vi "Anti-Tip.vi"() -> ()   [LabVIEW 2014]
uses:
  Begin/Global RefNums.vi
  Begin/Global Variables.vi
  _Dependencies/NavX/navX-MXP IMU.lvlib
panel:
  in  "Min Roll":dbl=-12.0
  in  "Min Pitch":dbl=-9.0
  in  "Max Roll":dbl=7.0
  in  "Max Pitch":dbl=6.0
  in  "Buffer":dbl=5.0
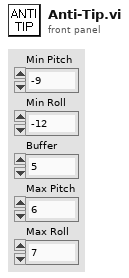
[diagram p1: front panel]
types:
  T1 = typedef "navX-MXP IMU.lvlib/navX Device TypeDef.ctl" = cluster{"navX Interface Protocol":T2, "navX Interface Protocol TypeDefs":cluster{"SPIDevRef":T3, "I2CDevRef":T6}, "navX System Information":cluster{"Board Information":T8, "Status":T9, "Offsets":T13}, "navX Common Information":cluster{"Update Rate (4Hz-60Hz)":T14, "refnum name":string, "error":errorcluster}}
  T2 = typedef "navX-MXP IMU.lvlib/navX Interface Protocol.ctl" = enum16{"SPI", "I2C"}
  T3 = typedef "WPI_SPIDevRef.ctl" = cluster{"DevStatus":errorcluster, "Handle":i32, "Controller":T4, "SPI Bus":T5}
  T4 = typedef "FPGA_TypedefDigitalModule.ctl" = enum16{"Controller 1"}
  T5 = typedef "spi_bus.ctl" = enum16{"SPI On-Board, CS0", "SPI On-Board, CS1", "SPI On-Board, CS2", "SPI On-Board, CS3", "SPI MXP", "Invalid"}
  T6 = typedef "WPI_I2CDevRef.ctl" = cluster{"DevStatus":errorcluster, "Controller":T4, "Device Address":u8, "Handle":i32, "I2C Bus":T7}
  T7 = typedef "i2c_bus.ctl" = enum16{"I2C On-Board", "I2C MXP", "Invalid"}
  T8 = typedef "navX-MXP IMU.lvlib/navX Board Information.ctl" = cluster{"WhoAmI (50 | 0x32)":u8, "Board Revision":u8, "Firmware Major Version":u8, "Firmware Minor Version":u8}
  T9 = typedef "navX-MXP IMU.lvlib/navX Status Data.ctl" = cluster{"Update Rate Hz":u8, "Accelerometer Full-Scale Range":u8, "Gyro Full-Scale Range":u16, "NAVX_OP_STATUS":T10, "NAVX_CAL_STATUS":T11, "NAVX_SELFTEST_STATUS":u8, "NAVX_SENSOR_STATUS":T12}
  T10 = typedef "navX-MXP IMU.lvlib/navX NAVX_OP_STATUS.ctl" = u8
  T11 = typedef "navX-MXP IMU.lvlib/navX NAVX_CAL_STATUS.ctl" = u8
  T12 = typedef "navX-MXP IMU.lvlib/navX NAVX_SENSOR_STATUS.ctl" = cluster{"MOVING":bool, "YAW_STABLE":bool, "MAG_DISTURBANCE":bool, "ALTITUDE_VALID":bool, "SEALEVEL_PRESS_SET":bool, "FUSED_HEADING_VALID":bool}
  T13 = typedef "navX-MXP IMU.lvlib/navX Offsets Data.ctl" = cluster{"Yaw":dbl, "Quat W":dbl, "Quat X":dbl, "Quat Y":dbl, "Quat Z":dbl}
  T14 = typedef "navX-MXP IMU.lvlib/navX Update Rate.ctl" = u8
  T15 = typedef "navX-MXP IMU.lvlib/navX YPRH Data.ctl" = cluster{"Yaw":dbl, "Pitch":dbl, "Roll":dbl, "Heading":dbl}
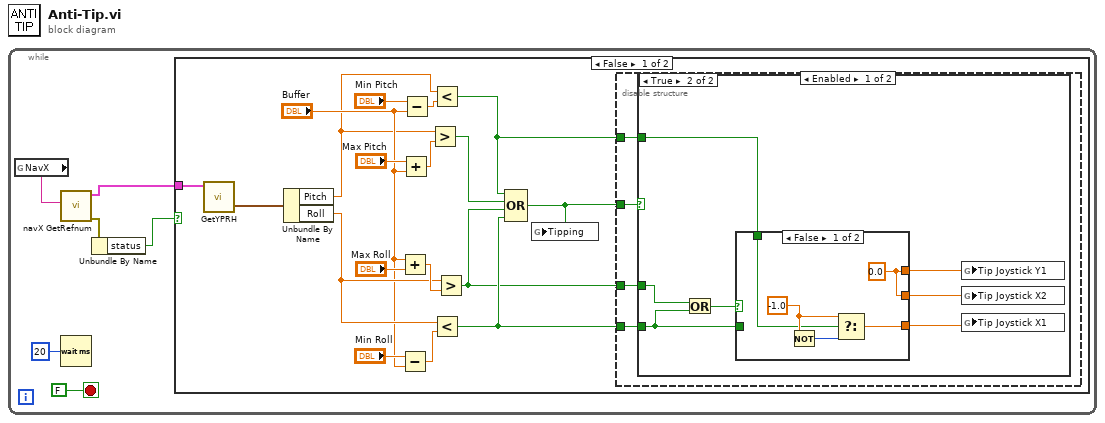
[diagram p0: block diagram]
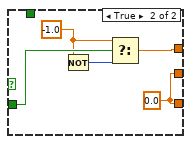
[diagram p3: hidden frame]
diagram:
  n1 = while {
    stop <- FALSE stop-if-true
    n2 = global read "Global RefNums.vi" "NavX"() -> (w4:string)
    n3 = call "navX GetRefnum.vi"("refnum name"=w4) -> ("error out"=w2:errorcluster, "navX Device TypeDef"=w3:T1)  [unwired: 9 in]
    n4 = Wait (ms)(milliseconds to wait=u32 20) -> ()  [unwired: 1 out]
    n5 = Unbundle By Name(w2) -> ("status"=w1:bool)
    n6 = case shown="False" w1 {
      tunnel: w3 -> [w7 _]
      frame False {
        n7 = call "GetYPRH.vi"("navX Device TypeDef"=w7) -> ("YPRH"=w10:T15)  [unwired: 8 in, 2 out]
        n8 = Unbundle By Name(w10) -> ("Pitch"=w13:dbl, "Roll"=w20:dbl)
        n9 = Add(x="Buffer", y="Max Roll") -> (x+y=w21:dbl)
        n10 = Subtract(x="Min Roll", y="Buffer") -> (x-y=w19:dbl)
        n11 = Add(x="Max Pitch", y="Buffer") -> (x+y=w22:dbl)
        n12 = Subtract(x="Min Pitch", y="Buffer") -> (x-y=w15:dbl)
        n13 = Greater?(x=w13, y=w22) -> (0:w14:bool)
        n14 = Less?(x=w13, y=w15) -> (x < y?=w9:bool)
        n15 = Less?(x=w20, y=w19) -> (x < y?=w12:bool)
        n16 = Greater?(x=w20, y=w21) -> (0:w11:bool)
        n17 = Compound Arithmetic op=OR(w9, w14, w11, w12) -> (w8:bool)
        n18 = global write "Global Variables.vi" "Tipping"(w8) -> ()
        n19 = disable-structure shown="Enabled" {
          disable-tunnel: w8 -> [w28 _]
          disable-tunnel: w12 -> [w27 _]
          disable-tunnel: w11 -> [w26 _]
          disable-tunnel: w9 -> [w25 _]
          frame Enabled {
            n20 = case shown="True" w28 {
              tunnel: w27 -> [_ w33]
              tunnel: w26 -> [_ w35]
              tunnel: w25 -> [_ w29]
              frame False {
              }
              frame True {
                n21 = Or(x=w35, y=w33) -> (x .or. y?=w34:bool)
                n22 = case shown="False" w34 {
                  tunnel: w33 -> [_ w45]
                  tunnel: [w36 w42] -> w32
                  tunnel: [w37 w42] -> w31
                  tunnel: [w37 w41] -> w30
                  tunnel: w29 -> [w38 _]
                  frame False {
                    w40 = -1.0 ("t")
                    w37 = 0.0 ("t")
                    n23 = Not(x=w40) -> (.not. x?=w39:u32)
                    n24 = Select(t=w40, s=w38, f=w39) -> (s? t:f=w36:dbl)
                  }
                  frame True {
                    w42 = 0.0 ("t")
                    w44 = -1.0 ("t")
                    n25 = Not(x=w44) -> (.not. x?=w43:u32)
                    n26 = Select(t=w44, s=w45, f=w43) -> (s? t:f=w41:dbl)
                  }
                }
                n27 = global write "Global Variables.vi" "Tip Joystick Y1"(w30) -> ()
                n28 = global write "Global Variables.vi" "Tip Joystick X2"(w31) -> ()
                n29 = global write "Global Variables.vi" "Tip Joystick X1"(w32) -> ()
              }
            }
          }
          frame Disabled {
          }
        }
      }
      frame True {
      }
    }
  }
